vi "Global Log Filter Example - Filter From Subscriber(Queue).vi"() -> ()   [LabVIEW 2017]
uses:
  user.lib/_NEVSTOP/Communicable State Machine(CSM)/_Support/Typedef/_CSM_GlobalLog Filter Rules - v1.0.ctl
  user.lib/_NEVSTOP/Communicable State Machine(CSM)/_Support/Typedef/_CSM_GlobalLog_MSG_TYPE.ctl
  user.lib/_NEVSTOP/Communicable State Machine(CSM)/_Support/Typedef/_CSM_GlobalLog_STATE_TYPE.ctl
  user.lib/_NEVSTOP/Communicable State Machine(CSM)/Utility/_support/Periodic String Filter Level.ctl
  user.lib/_NEVSTOP/Communicable State Machine(CSM)/Utility/Periodic String Filter Setting.ctl
  user.lib/_NEVSTOP/Communicable State Machine(CSM)/_Support/GlobalEvent/GEvt-Filter Global Log - v1.0.vi
  1. Create a reuse Module/1. Create a reuse Module.lvlib
  user.lib/_NEVSTOP/Communicable State Machine(CSM)/Communicable State Machine.lvlib
  user.lib/_NEVSTOP/Communicable State Machine(CSM)/_Shared/CSM Shared.lvlib
panel:
  out "LogInQ":i32
  out "State History 2":string
  out "log handling Speed(#/s)":dbl
  out "Backlog Change(#/s)":dbl
  out "Level":T1
  in  "Stop":bool
  in  "Rules-v1":T2={"Global"={"CSM"=["Module2"], "LogType"=[], "State"=[], "StateType"=[]}, "CSM"={"LogType"=[{"CSM"="Module1", "LogType"=enum."State Change"}], "State"=[{"CSM"="Module3", "State"=""}], "StateType"=[]}}
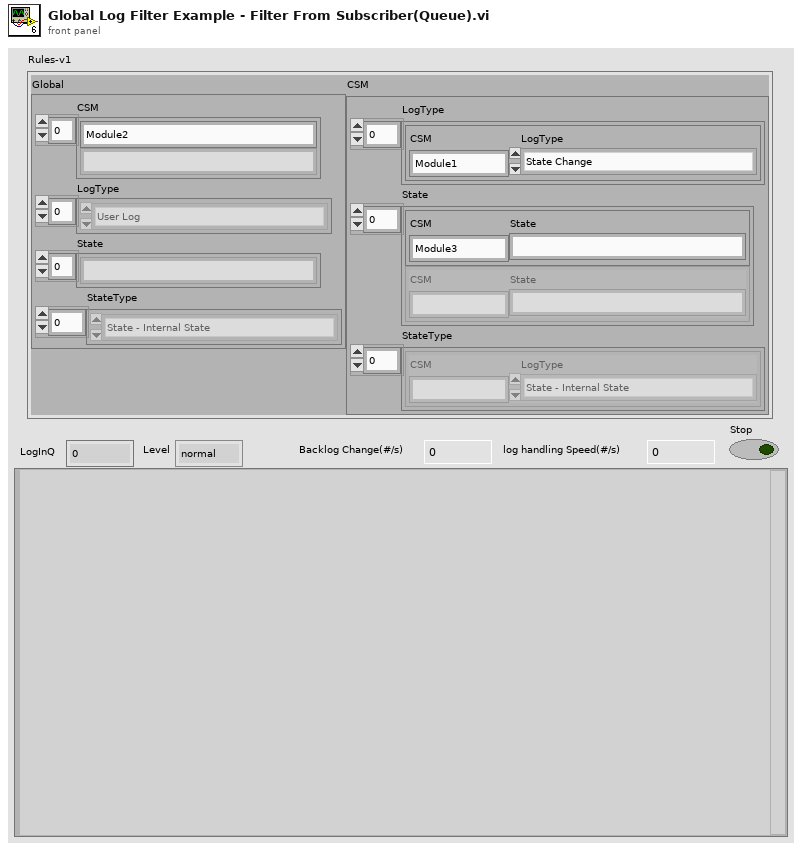
[diagram p1: front panel]
types:
  T1 = typedef "Communicable State Machine.lvlib/Periodic String Filter Level.ctl" = enum16{"normal", "L1", "L2", "L3", "L4"}
  T2 = typedef "Communicable State Machine.lvlib/_CSM_GlobalLog Filter Rules - v1.0.ctl" = cluster{"Global":cluster{"CSM":string[], "LogType":T3[], "State":string[], "StateType":T4[]}, "CSM":cluster{"LogType":cluster{"CSM":string, "LogType":T3}[], "State":cluster{"CSM":string, "State":string}[], "StateType":cluster{"CSM":string, "LogType":T4}[]}}
  T3 = typedef "Communicable State Machine.lvlib/_CSM_GlobalLog_MSG_TYPE.ctl" = enum16{"User Log", "State Change", "Status", "Interrupt", "Register", "Unregister", "Error Log", "Module Created", "Module Destroyed"}
  T4 = typedef "Communicable State Machine.lvlib/_CSM_GlobalLog_STATE_TYPE.ctl" = enum16{"State - Internal State", "State - External Message", "State - Response", "State - Complete"}
  T5 = typedef "Communicable State Machine.lvlib/Periodic String Filter Setting.ctl" = cluster{"threashold(#/s)":dbl, "Check Peroid(s)":dbl}
  T6 = typedef "Communicable State Machine.lvlib/_CSM_GlobalLog_MSG.ctl" = cluster{"Name (\"\" to Use UUID)":string, "Current State":string, "Arguments":string, "Source Message":T7, "Source Module":string, "Complete(T)/Start(F)":bool, "LogType":T3, "Time Stamp":timestamp}
  T7 = typedef "Communicable State Machine.lvlib/_CSM_Response Source Message.ctl" = cluster{"‘State":string, "’Arguments":string, "’Error":errorcluster}
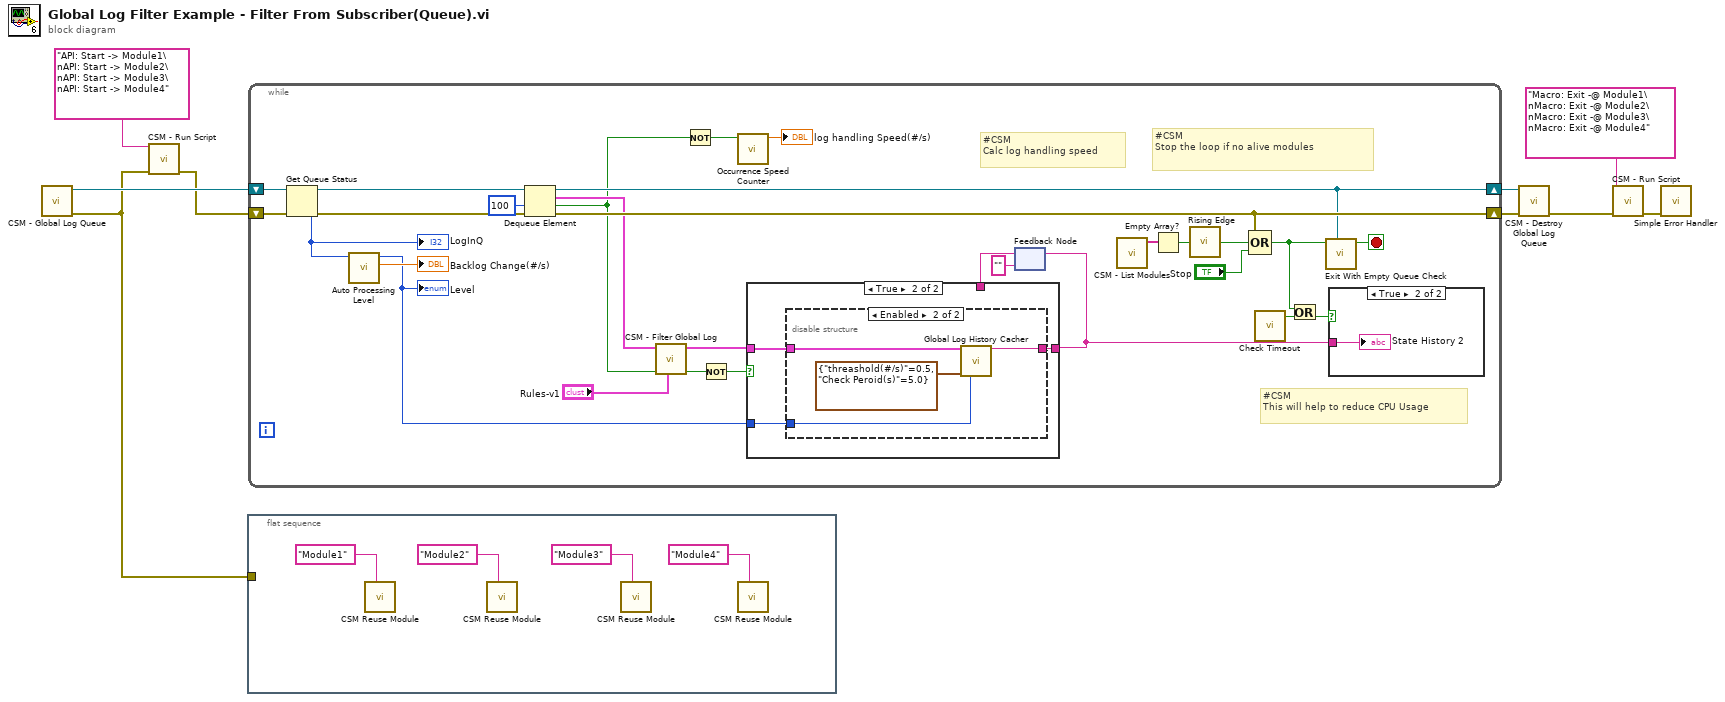
[diagram p0: block diagram]
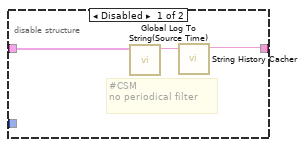
[diagram p3: hidden frame]
diagram:
  n1 = call "CSM - Global Log Queue.vi"() -> ("error out"=w4:errorcluster, "GlobalEvent Queue"=w7:refnum<queue>)  [unwired: 10 in]
  n2 = call "CSM - Run Script.vi"("CSM Scripts"="API: Start -> Module1\nAPI: Start -> Module2\nAPI: Start -> Module3\nAPI: Start -> Module4" ("single-line text"), "error in (no error)"=w4) -> ("error out"=w5:errorcluster)  [unwired: 11 in, 2 out]
  n3 = flat-sequence {
    tunnel: w4 -> [_]
    frame #0 {
      n4 = call "CSM Reuse Module.vi"("Name (\"\" to Use UUID)"="Module1" ("Name(\"\" to use uuid)")) -> ()  [unwired: 11 in]
      n5 = call "CSM Reuse Module.vi"("Name (\"\" to Use UUID)"="Module2" ("Name(\"\" to use uuid)")) -> ()  [unwired: 11 in]
      n6 = call "CSM Reuse Module.vi"("Name (\"\" to Use UUID)"="Module3" ("Name(\"\" to use uuid)")) -> ()  [unwired: 11 in]
      n7 = call "CSM Reuse Module.vi"("Name (\"\" to Use UUID)"="Module4" ("Name(\"\" to use uuid)")) -> ()  [unwired: 11 in]
    }
  }
  n8 = while {
    shift-right: [w41] -> w9
    shift-left: w5 -> [w38]
    shift-right: [w27] -> w8
    shift-left: w7 -> [w42]
    stop <- w28 stop-if-true
    # "#CSM\nCalc log handling speed"
    # "#CSM\nStop the loop if no alive modules"
    # "#CSM\nThis will help to reduce CPU Usage"
    n9 = Get Queue Status(queue=w42, error in (no error)=w38) -> (queue out=w40:refnum<queue>, error out=w39:errorcluster, # elements in queue=w23:i32)  [unwired: 1 in, 5 out]
    "LogInQ" <- w23
    n10 = call "Auto Processing Level.vi"("#Left In Q"=w23) -> ("LogInQ Changing Speed (#/s)"=→"Backlog Change(#/s)":dbl, "Level"=w22:T1)  [unwired: 8 in, 1 out]
    "Level" <- w22
    n11 = Dequeue Element(queue=w40, timeout in ms (-1)=100, error in (no error)=w39) -> (queue out=w27:refnum<queue>, element=w19:T6, timed out?=w14:bool, error out=w41:errorcluster)
    n12 = call-poly "CSM - Filter Global Log.vi"("Rules-v1"="Rules-v1", "Matched Previous?"=w14, "Cross CSM Data (In)"=w19) -> ("Matched? (Dup)"=w17:bool, "Cross CSM Data"=w18:T6)  [unwired: 7 in]
    n13 = Not(x=w14) -> (.not. x?=w16:bool)
    n14 = Not(x=w17) -> (.not. x?=w15:bool)
    n15 = call "Occurrence Speed Counter.vi"("Occured? (T)"=w16) -> ("Speed (#/s)"=→"log handling Speed(#/s)":dbl)  [unwired: 8 in, 2 out]
    n16 = feedback #1("" ("String Cache")) -> (w34:string)
    n17 = case shown="True" w15 {
      tunnel: w18 -> [_ w46]
      tunnel: [w43 w45] -> w35
      tunnel: w34 -> [w43 _]
      tunnel: w22 -> [_ w44]
      frame False {
      }
      frame True {
        n18 = disable-structure shown="Enabled" {
          disable-tunnel: w46 -> [w49 w52]
          disable-tunnel: [w47 w53] -> w45
          disable-tunnel: w44 -> [_ w51]
          frame Disabled {
            # "#CSM \nno periodical filter"
            n19 = call "Global Log To String(Source Time).vi"("Log"=w49) -> ("Log String"=w48:string)  [unwired: 9 in]
            n20 = call "String History Cacher.vi"("String"=w48) -> ("String Cache"=w47:string)  [unwired: 10 in]
          }
          frame Enabled {
            n21 = call "Global Log History Cacher.vi"("Cross CSM Data"=w52, "Settings"=T5 {"threashold(#/s)"=0.5, "Check Peroid(s)"=5.0}, "Level (Normal)"=w51) -> ("String Cache"=w53:string)  [unwired: 12 in]
          }
        }
      }
    }
    n22 = feedback-in #1(w35) -> ()
    n23 = call "CSM - List Modules.vi"() -> ("Module Names"=w33:string[])  [unwired: 10 in, 1 out]
    n24 = Empty Array?(array=w33) -> (empty?=w32:bool)
    n25 = call "Rising Edge.vi"("Signal"=w32) -> ("Rising Edge"=w31:bool)
    n26 = Compound Arithmetic op=OR(w41, w31, "Stop") -> (w25:bool)
    n27 = call "Check Timeout.vi"() -> ("Timeout"=w36:bool)  [unwired: 8 in]
    n28 = Or(x=w25, y=w36) -> (x .or. y?=w26:bool)
    n29 = call "Exit With Empty Queue Check.vi"("Queue"=w27, "Stop"=w25) -> ("Exit"=w28:bool)  [unwired: 8 in, 1 out]
    n30 = case shown="True" w26 {
      tunnel: w35 -> [_ w54]
      frame False {
      }
      frame True {
        "State History 2" <- w54
      }
    }
  }
  n31 = call "CSM - Destroy Global Log Queue.vi"("Error In"=w9, "Global Log Queue"=w8) -> ("error out"=w2:errorcluster)  [unwired: 9 in]
  n32 = call "CSM - Run Script.vi"("CSM Scripts"="Macro: Exit -@ Module1\nMacro: Exit -@ Module2\nMacro: Exit -@ Module3\nMacro: Exit -@ Module4" ("single-line text"), "error in (no error)"=w2) -> ("error out"=w1:errorcluster)  [unwired: 11 in, 2 out]
  n33 = call <vilib>:"Simple Error Handler.vi"("error in (no error)"=w1) -> ()  [unwired: 4 in, 5 out]
